vi "Actor Core.vi"(8 "error in":errorcluster, 11 "Lutron QS Object in":refnum<class "Lutron QS Object.lvclass">) -> (0 "error out":errorcluster, 3 "Actor out":refnum<class "Actor.lvclass">)   [LabVIEW 2014]
doc: "(<B>Filename</B>: Actor Framework.lvlib:Actor.lvclass:Actor Core.vi)\n\nReceives messages to the actor, reacts to them, and initiates any error handling that may shut the actor down.\n\nDescendant classes may override this VI to append parallel tasks for the actor to complete while it handles messages. Overrides use the Call Parent Method node."
uses:
  <vilib>/ActorFramework/Actor/Actor.lvclass
  Lutron QS Object.lvclass
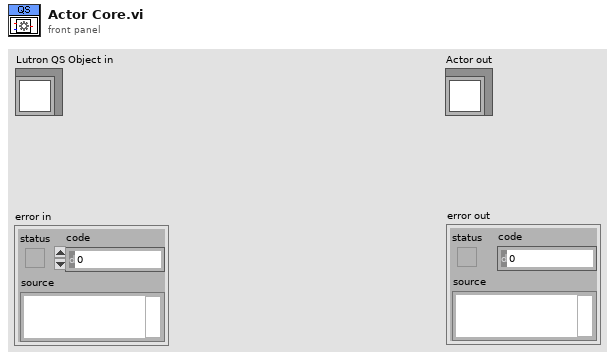
[diagram p1: front panel]
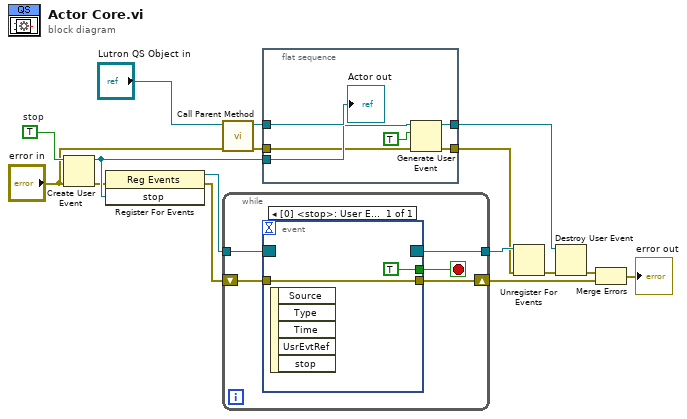
[diagram p0: block diagram]
diagram:
  w13 = TRUE  # stop
  n1 = Create User Event(user event datatype=w13, error in="error in") -> (user event=w9:refnum<user-event>, error out=w6:errorcluster)
  n2 = register-events(error in=w6, w9) -> (reference out=w12:refnum<event-registration>, error out=w4:errorcluster)  [unwired: 1 in]
  n3 = call-parent "Call Parent Method"("error in"="error in", "Actor in"="Lutron QS Object in") -> ("error out"=w16:errorcluster, "Actor out"=w15:refnum<class "Actor.lvclass">)  [unwired: 8 in]
  n4 = while {
    tunnel: w12 -> [w21]
    tunnel: [w19] -> w11
    shift-right: [w17] -> w2
    shift-left: w4 -> [w18]
    stop <- w20 stop-if-true
    n5 = event shown="[0] <stop>: User Event" {
      selector: w21 -> [_]
      dyn-events: [_] -> w19
      timeout: _ -> [_]
      tunnel: [TRUE] -> w20
      tunnel: w18 -> [w22]
      tunnel: [w22] -> w17
      event User Event {
        n6 = event-data() -> ()  [unwired: 1 in, 5 out]
      }
    }
  }
  n7 = flat-sequence {
    tunnel: w16 -> [w26]
    tunnel: w15 -> [w29]
    tunnel: w9 -> [w28]
    tunnel: [w27] -> w8
    tunnel: [w25] -> w7
    frame #0 {
      n8 = Generate User Event(user event=w28, event data cluster=TRUE ("event data"), error in=w26) -> (user event out=w27:refnum<user-event>, error out=w25:errorcluster)  [unwired: 1 in]
      "Actor out" <- w29
    }
  }
  n9 = Unregister For Events(event registration refnum=w11, error in=w7) -> (error out=w10:errorcluster)
  n10 = Destroy User Event(user event=w8, error in=w10) -> (error out=w3:errorcluster)
  n11 = Merge Errors(w3, w2) -> (→"error out":errorcluster)
